vi "New.vi"(8 "error in (no error)":errorcluster, 10 "Secret":string) -> (0 "error out":errorcluster, 3 "TicketAuthentactor out":refnum<class "TicketAuthentactor.lvclass">)   [LabVIEW 2020, in "wamplv.lvlib" / "TicketAuthentactor.lvclass"]
uses:
  TicketAuthentactor.lvclass
  TicketAuthentactor.lvclass/TicketAuthentactor.ctl
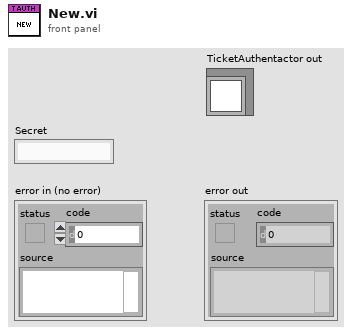
[diagram p1: front panel]
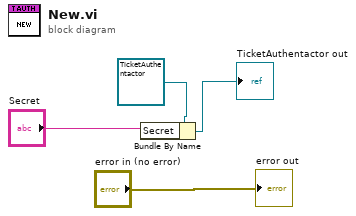
[diagram p0: block diagram]
diagram:
  n1 = Bundle By Name(cluster=refnum<class "TicketAuthentactor.lvclass"> refnum ("wamplv.lvlib:TicketAuthentactor.lvclass"), "Secret"="Secret") -> (→"TicketAuthentactor out":refnum<class "TicketAuthentactor.lvclass">)
  "error out" <- "error in (no error)"
